vi "Add to Project.vi"(8 "error in (no error)":errorcluster, 11 "Abstract Message Scripter in":refnum<class "Abstract Message Scripter.lvclass">) -> (0 "error out":errorcluster, 3 "Abstract Message Scripter out":refnum<class "Abstract Message Scripter.lvclass">)   [LabVIEW 2020, in "Message Maker.lvlib" / "Abstract Message Scripter.lvclass"]
uses:
  Abstract Message Scripter.lvclass
  Message Scripter/Message Scripter.lvclass
  Message Maker.lvlib
  _support/Localized Strings.vi
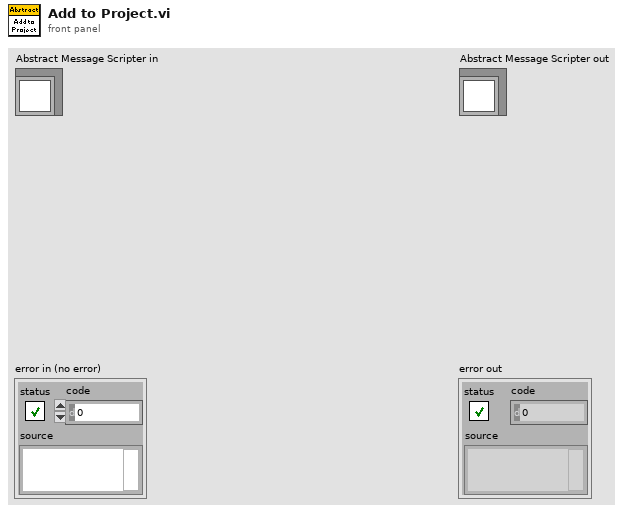
[diagram p1: front panel]
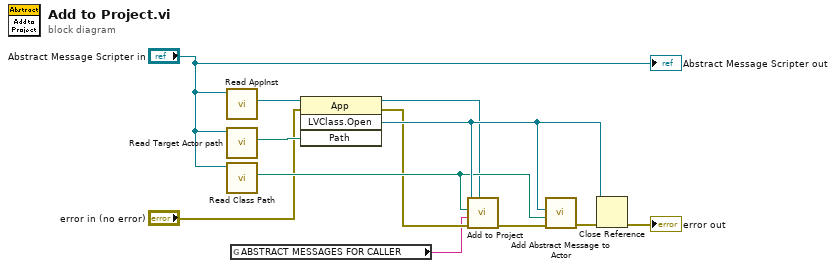
[diagram p0: block diagram]
diagram:
  n1 = call "Read AppInst.vi"("Message Maker in"="Abstract Message Scripter in") -> ("AppInst"=w5:refnum<vi>)  [unwired: 10 in]
  n2 = call "Read Target Actor path.vi"("Message Scripter in"="Abstract Message Scripter in") -> ("Target Actor path"=w12:path)  [unwired: 10 in]
  n3 = call "Read Class Path.vi"("Message Scripter in"="Abstract Message Scripter in") -> ("Class Path"=w8:path)  [unwired: 10 in]
  n4 = global read "Localized Strings.vi" "ABSTRACT MESSAGES FOR CALLER"() -> (w1:string)
  n5 = invoke class="App" method="LVClass.Open"(reference=w5, error in="error in (no error)", "Path"=w12) -> (reference out=w2:refnum<vi>, error out=w7:errorcluster, "LVClass.Open"=w9:refnum<vi>)  [unwired: 1 in, 1 out]
  n6 = call "Add to Project.vi"("AppInst"=w2, "error in (no error)"=w7, "Folder"=w1, "Class Path"=w8, "Actor"=w9) -> ("error out"=w10:errorcluster)  [unwired: 6 in]
  n7 = call "Add Abstract Message to Actor.vi"("error in (no error)"=w10, "Abstract Message Path"=w8, "Target Actor in"=w9) -> ("error out"=w11:errorcluster)  [unwired: 8 in]
  n8 = Close Reference(reference=w9, error in (no error)=w11) -> (error out=→"error out":errorcluster)
  "Abstract Message Scripter out" <- "Abstract Message Scripter in"
